vi "TDMSFindGroupChannel.vi"(5 "groups/channels in file":string[][](array[string]), 7 "Tracenr":i32, 8 "Group in":string, 9 "channels in":string[](array[string])) -> (1 "#Channels":i32, 2 "Groups out":string[](array[string]), 3 "Channels out":string[](array[string]))   [LabVIEW 2018]
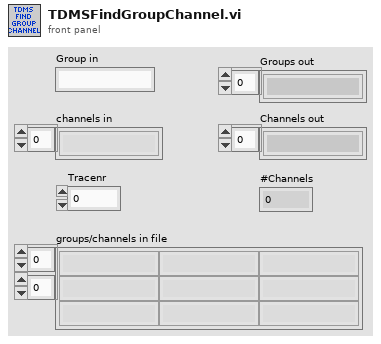
[diagram p1: front panel]
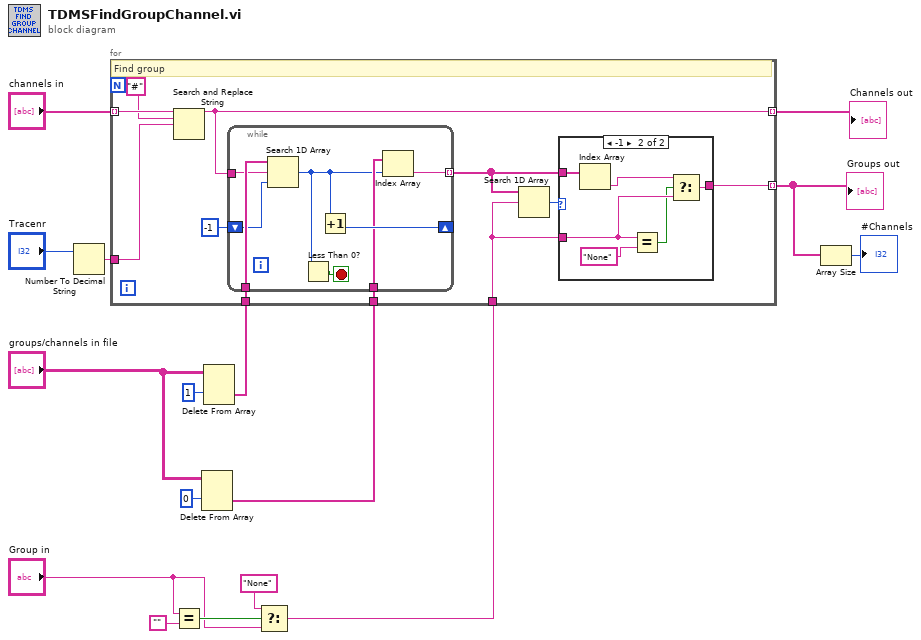
[diagram p0: block diagram]
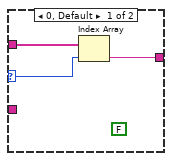
[diagram p2: hidden frame]
diagram:
  n1 = Number To Decimal String(number="Tracenr") -> (decimal integer string=w11:string)  [unwired: 1 in]
  n2 = Equal?(x="Group in", y="") -> (x = y?=w4:bool)
  n3 = Delete From Array(array="groups/channels in file", index (row)=0) -> (deleted portion=w16:string[])  [unwired: 2 in, 1 out]
  n4 = Delete From Array(array="groups/channels in file", index (row)=1) -> (deleted portion=w15:string[])  [unwired: 2 in, 1 out]
  n5 = Select(t="None", s=w4, f="Group in") -> (s? t:f=w1:string)
  n6 = for {
    tunnel: "channels in" -> [w27] mode=indexing
    tunnel: [w23] -> w14 mode=indexing
    tunnel: w11 -> [w25]
    tunnel: w15 -> [w24]
    tunnel: w16 -> [w21]
    tunnel: [w19] -> w7 mode=indexing
    tunnel: w1 -> [w18]
    # "Find group"
    n7 = Search and Replace String(input string=w27, search string="#" ("substring (\"\")"), replace string=w25) -> (result string=w23:string)  [unwired: 5 in, 3 out]
    n8 = while {
      tunnel: w24 -> [w44]
      tunnel: w23 -> [w43]
      shift-right: [w40] -> _
      shift-left: -1 ("index of element") -> [w41]
      tunnel: w21 -> [w39]
      tunnel: [w37] -> w20 mode=indexing
      stop <- w42 stop-if-true
      n9 = Search 1D Array(1D array=w44, element=w43, start index (0)=w41) -> (index of element=w38:i32)
      n10 = Less Than 0?(x=w38) -> (x < 0?=w42:bool)
      n11 = Increment(x=w38) -> (x+1=w40:i32)
      n12 = Index Array(array=w39, index=w38) -> (element=w37:string)
    }
    n13 = Search 1D Array(1D array=w20, element=w18) -> (index of element=w17:i32)  [unwired: 1 in]
    n14 = case shown="-1" w17 {
      selector: w17 -> [w28 _]
      tunnel: w20 -> [w30 w36]
      tunnel: [w29 w33] -> w19
      tunnel: w18 -> [_ w34]
      frame 0, Default {
        (unwired) FALSE
        n15 = Index Array(array=w30, index=w28) -> (element=w29:string)
      }
      frame -1 {
        n16 = Index Array(array=w36) -> (element=w35:string)  [unwired: 1 in]
        n17 = Equal?(x=w34, y="None") -> (x = y?=w32:bool)
        n18 = Select(t=w35, s=w32, f=w34) -> (s? t:f=w33:string)
      }
    }
  }
  "Channels out" <- w14
  "Groups out" <- w7
  n19 = Array Size(array=w7) -> (size(s)=→"#Channels":i32)
